vi "rtime.vi"() -> ()   [LabVIEW 2017]
panel:
  in  "Slide 3":dbl(slide) scale=-200.0..200.0
  in  "Slide 2":dbl(slide) scale=-200.0..200.0
  in  "Slide":dbl(slide) scale=-200.0..200.0
  in  "Channel Name 4":tag
  in  "Channel Name 3":tag
  in  "Channel Name 2":tag
  in  "stop":bool
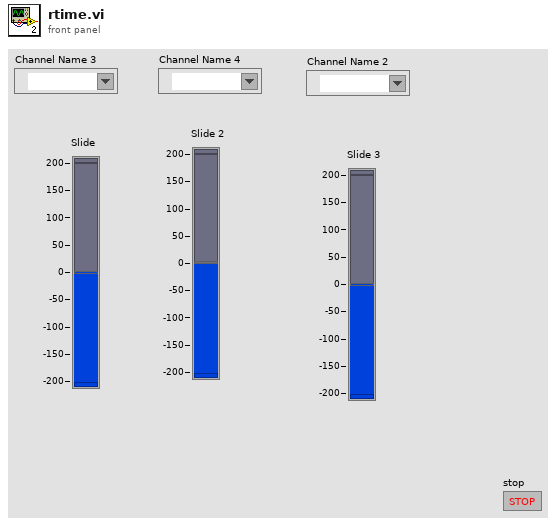
[diagram p1: front panel]
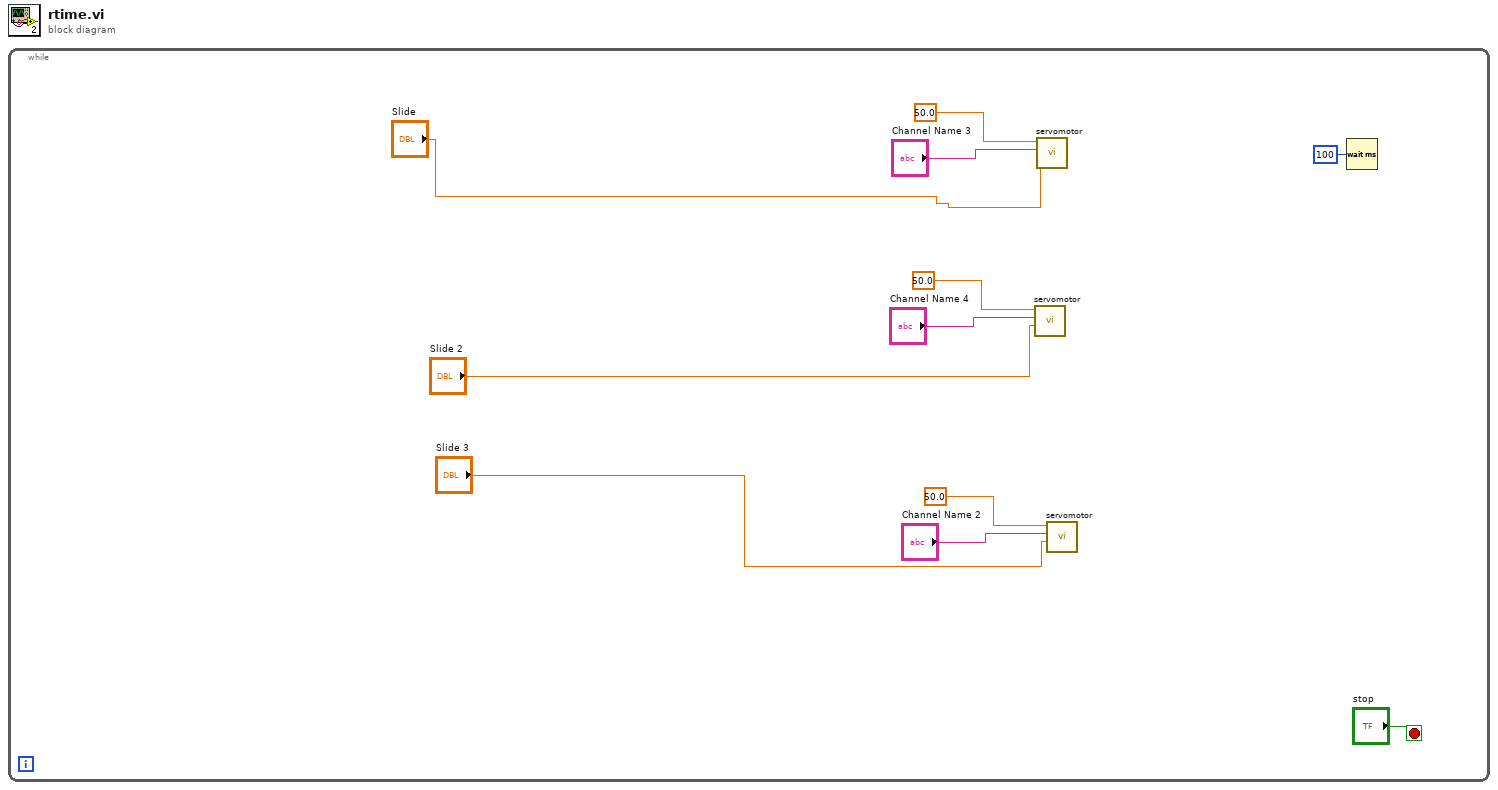
[diagram p0: block diagram]
diagram:
  n1 = while {
    stop <- "stop" stop-if-true
    n2 = call "servomotor.vi"("posicion"="Slide 2", "Channel Name"="Channel Name 4", "Frequency [Hz]"=50.0) -> ()  [unwired: 9 in]
    n3 = call "servomotor.vi"("posicion"="Slide", "Channel Name"="Channel Name 3", "Frequency [Hz]"=50.0) -> ()  [unwired: 9 in]
    n4 = call "servomotor.vi"("posicion"="Slide 3", "Channel Name"="Channel Name 2", "Frequency [Hz]"=50.0) -> ()  [unwired: 9 in]
    n5 = Wait (ms)(milliseconds to wait=u32 100) -> ()  [unwired: 1 out]
  }
